vi "Execute.vi"(5 "Init user event out":refnum<user-event>, 7 "user event in":refnum<user-event>, 8 "Advanced Waveform In":refnum<class "Advanced Waveform.lvclass">, 9 "Waveform Type Message in":refnum<class "Waveform Type Message.lvclass">, 10 "Command Queue":refnum<queue>, 11 "error in (no error)":errorcluster) -> (0 "Advanced Waveform Out":refnum<class "Advanced Waveform.lvclass">, 1 "Waveform Type Message out":refnum<class "Waveform Type Message.lvclass">, 2 "Stop":bool, 3 "error out":errorcluster)   [LabVIEW 2011, in "Waveform Type Message.lvclass"]
uses:
  Waveform Type Message.lvclass
  Advanced Waveform Class/Advanced Waveform.lvclass
  Message.lvclass
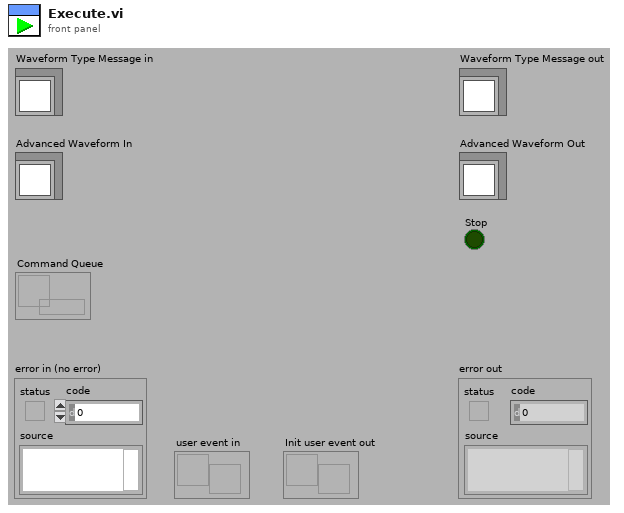
[diagram p1: front panel]
types:
  T1 = typedef "Waveform Type.ctl" = enum16{"Sine", "Square", "Triangle"}
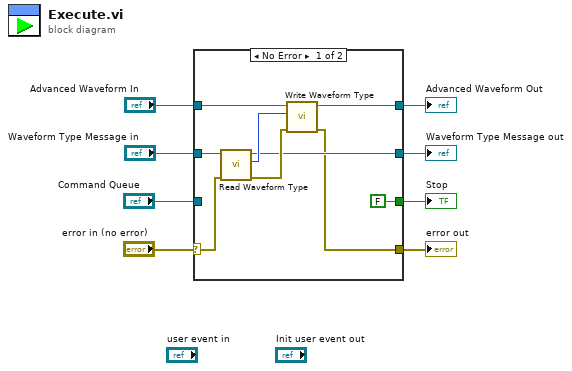
[diagram p0: block diagram]
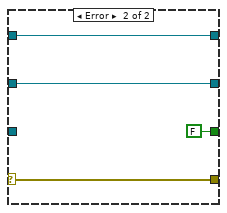
[diagram p2: hidden frame]
diagram:
  n1 = case shown="No Error" "error in (no error)" {
    selector: "error in (no error)" -> [w16 w18]
    tunnel: [w10 w18] -> w7
    tunnel: "Advanced Waveform In" -> [w15 w21]
    tunnel: "Waveform Type Message in" -> [w17 w20]
    tunnel: [w12 w20] -> w4
    tunnel: [w11 w21] -> w3
    tunnel: [FALSE FALSE] -> w2
    tunnel: "Command Queue" -> [_ _]
    frame No Error {
      n2 = call-dynamic "Read Waveform Type.vi"("error in (no error)"=w16, "Waveform Type Message in"=w17) -> ("error out"=w14:errorcluster, "Waveform Type"=w13:T1, "Waveform Type Message out"=w12:refnum<class "Waveform Type Message.lvclass">)  [unwired: 7 in]
      n3 = call-dynamic "Write Waveform Type.vi"("error in (no error)"=w14, "Waveform Type"=w13, "Advanced Waveform in"=w15) -> ("error out"=w10:errorcluster, "Advanced Waveform out"=w11:refnum<class "Advanced Waveform.lvclass">)  [unwired: 7 in]
    }
    frame Error {
    }
  }
  "error out" <- w7
  "Waveform Type Message out" <- w4
  "Stop" <- w2
  "Advanced Waveform Out" <- w3
